vi "Pre-Init.vi"(8 "error in (no error)":errorcluster, 11 "Lockin Digitizer Driver in":refnum<class "Lockin Digitizer Driver.lvclass">) -> (0 "error out":errorcluster, 3 "Lockin Digitizer Driver out":refnum<class "Lockin Digitizer Driver.lvclass">)   [LabVIEW 2024, in "Lockin Digitizer Driver.lvclass"]
uses:
  Lockin Digitizer Driver.lvclass
  Pulse Driver.lvclass
  Lockin Digitizer Driver.lvclass/Lockin Digitizer Driver.ctl
  File/File Class/File.lvclass
panel:
  out "Lock-in channel indexes":i32[](array[numeric])
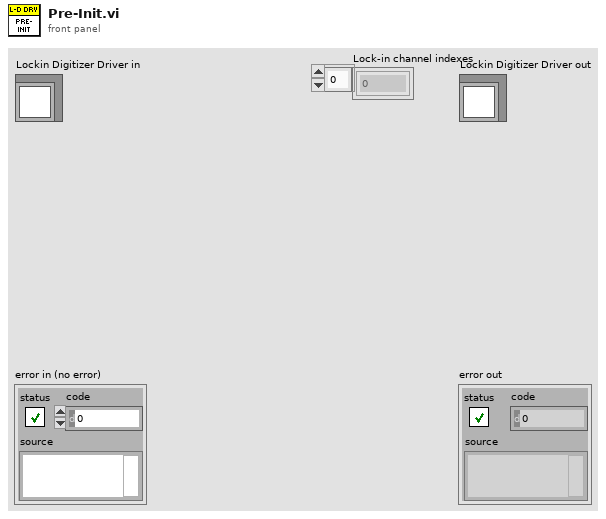
[diagram p1: front panel]
types:
  T1 = typedef "Lockin Digitizer Configuration.ctl" = cluster{"Post-trigger delay":dbl, "Post-trigger duration":dbl, "Rate":dbl, "Ranges":dbl[], "Re-name channels":string[], "Active channels":string, "External\nclock":bool, "Monitor time\nconstant":dbl, "Sync":bool, "Lock-in input channel phases":dbl[], "Output channels configuration":T2[]}
  T2 = typedef "Output Channel Configuration.ctl" = cluster{"Input channels":string, "Frequency":dbl, "Output amplitude":dbl, "Output channel number":i32}
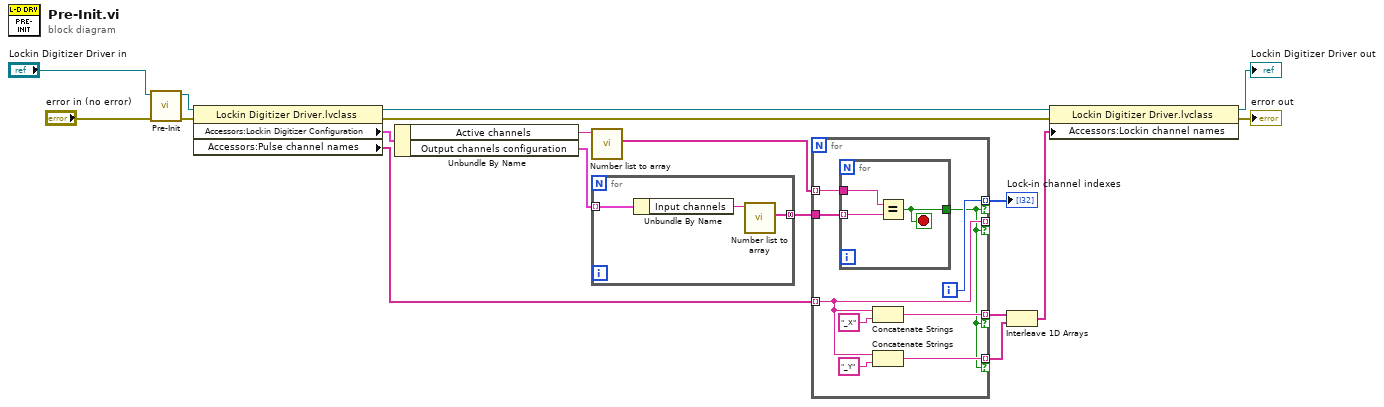
[diagram p0: block diagram]
diagram:
  n1 = call-parent "Pre-Init.vi"("error in (no error)"="error in (no error)", "Pulse Driver in"="Lockin Digitizer Driver in") -> ("error out"=w3:errorcluster, "Pulse Driver out"=w16:refnum<class "Lockin Digitizer Driver.lvclass">)  [unwired: 8 in]
  n2 = property class="Lockin Digitizer Driver.lvclass"(reference=w16, error in=w3) -> (reference out=w8:refnum<class "Lockin Digitizer Driver.lvclass">, error out=w7:errorcluster, "Accessors:Lockin Digitizer Configuration"=w15:T1, "Accessors:Pulse channel names"=w9:string[])
  n3 = Unbundle By Name(w15) -> ("Active channels"=w14:string, "Output channels configuration"=w13:T2[])
  n4 = call "Number list to array.vi"("Number list"=w14) -> ("Full names"=w11:string[])  [unwired: 7 in, 3 out]
  n5 = for {
    tunnel: w13 -> [w21] mode=indexing
    tunnel: [w20] -> w12 mode=concatenating
    n6 = Unbundle By Name(w21) -> ("Input channels"=w19:string)
    n7 = call "Number list to array.vi"("Number list"=w19) -> ("Full names"=w20:string[])  [unwired: 7 in, 3 out]
  }
  n8 = for {
    tunnel: w12 -> [w30]
    tunnel: w11 -> [w29] mode=indexing
    tunnel: [w28] -> w10 mode=indexing if=w22
    tunnel: w9 -> [w26] mode=indexing
    tunnel: [w26] -> _ mode=indexing if=w22
    tunnel: [w24] -> w6 mode=indexing if=w22
    tunnel: [w23] -> w5 mode=indexing if=w22
    i -> [w28]
    n9 = for {
      tunnel: w30 -> [w33] mode=indexing
      tunnel: w29 -> [w32]
      tunnel: [w31] -> w22
      stop <- w31 stop-if-true
      n10 = Equal?(x=w32, y=w33) -> (x = y?=w31:bool)
    }
    n11 = Concatenate Strings(w26, "_X" ("string")) -> (w24:string)
    n12 = Concatenate Strings(w26, "_Y" ("string")) -> (w23:string)
  }
  "Lock-in channel indexes" <- w10
  n13 = Interleave 1D Arrays(w6, w5) -> (w4:string[])
  n14 = property class="Lockin Digitizer Driver.lvclass"(reference=w8, error in=w7, "Accessors:Lockin channel names"=w4) -> (reference out=→"Lockin Digitizer Driver out":refnum<class "Lockin Digitizer Driver.lvclass">, error out=→"error out":errorcluster)
